vi "Export Routing and Faulting Custom Device.vi"(8 "error in":errorcluster, 9 "operation":T1(ring)=enum."replace or create with confirmation", 10 "datalog path (use dialog)":path, 11 "routing and faulting custom device in":T2 format="%.0x") -> (0 "error out":errorcluster, 3 "routing and faulting custom device out":T2 format="%.0x")   [LabVIEW 2017, in "Routing and Faulting Scripting.lvlib"]
uses:
  Routing and Faulting Scripting.lvlib
  <vilib>/NI Veristand/Custom Device API/Custom Device Item Ref.ctl
  <vilib>/NI/NI VeriStand Custom Device Import and Export Tool/ImportExport.lvlib
  <vilib>/NI Veristand/Custom Device API/Custom Device API.lvlib
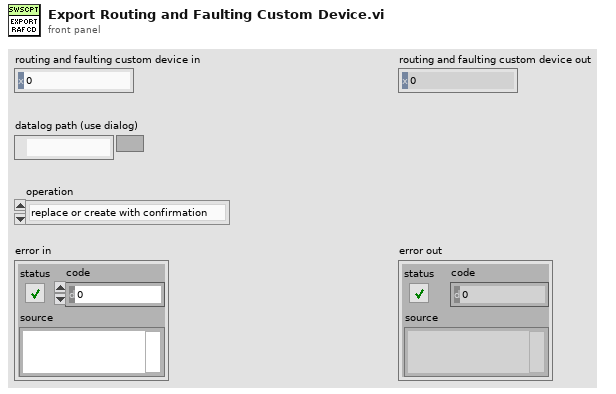
[diagram p1: front panel]
types:
  T1 = enum16{"open", "replace", "create", "open or create", "replace or create", "replace or create with confirmation"}
  T2 = typedef "Custom Device API.lvlib/Custom Device Item Ref.ctl" = u64
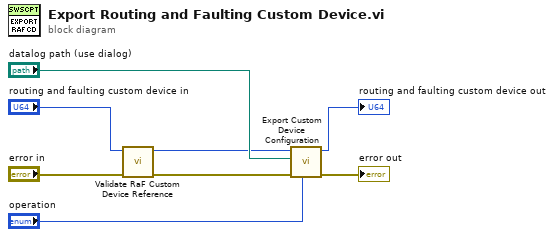
[diagram p0: block diagram]
diagram:
  n1 = call "Validate RaF Custom Device Reference.vi"("error in (no error)"="error in", "Routing and Faulting Custom Device Ref in"="routing and faulting custom device in") -> ("error out"=w3:errorcluster, "Routing and Faulting Custom Device Ref out"=w1:T2)  [unwired: 8 in]
  n2 = call <vilib>:"Export Custom Device Configuration.vi"("operation"="operation", "error in (no error)"=w3, "Path"="datalog path (use dialog)", "ID"=w1) -> ("error out"=→"error out":errorcluster, "ID out"=→"routing and faulting custom device out":u64)  [unwired: 6 in]
